vi "get_length_or_depth.vi"(8 "error in (no error)":errorcluster, 11 "ImageCollection in":refnum<class "ImageCollection.lvclass">) -> (0 "error out":errorcluster, 1 "total z depth":dbl[unit], 2 "movie length":dbl[unit], 3 "ImageCollection out":refnum<class "ImageCollection.lvclass">, 4 "type":T1)   [LabVIEW 2010, in "ImageCollection.lvclass"]
uses:
  ImageCollection.lvclass
  type_enum.ctl
  ImageCollection.lvclass/ImageCollection.ctl
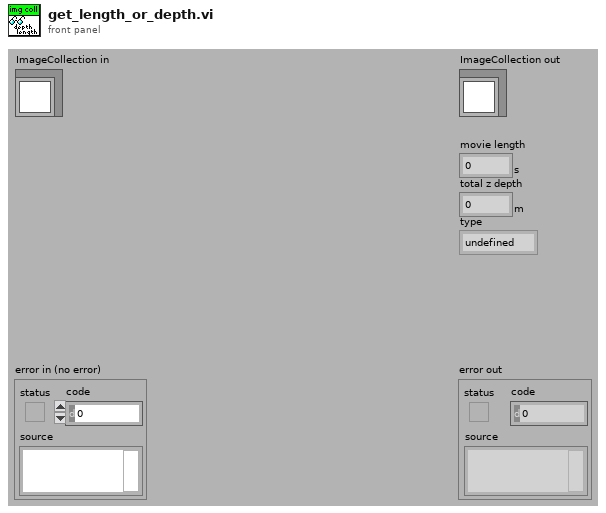
[diagram p1: front panel]
types:
  T1 = typedef "type_enum.ctl" = enum16{"undefined", "movie", "z-stack"}
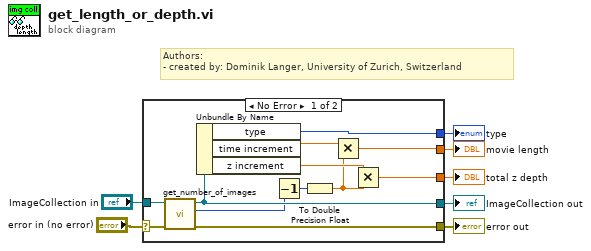
[diagram p0: block diagram]
diagram:
  # "Authors: \n- created by: Dominik Langer, University of Zurich, Switzerland"
  n1 = case shown="No Error" "error in (no error)" {
    selector: "error in (no error)" -> [w19 w21]
    tunnel: [w18 w21] -> w6
    tunnel: [w16 w20] -> w4
    tunnel: "ImageCollection in" -> [w17 w20]
    tunnel: [w10 _] -> w3
    tunnel: [w9 _] -> w2
    tunnel: [w8 _] -> w1
    frame No Error {
      n2 = call-dynamic "get_number_of_images.vi"("error in (no error)"=w19, "ImageCollection in"=w17) -> ("error out"=w18:errorcluster, "size"=w14:i32, "ImageCollection out"=w16:refnum<class "ImageCollection.lvclass">)  [unwired: 7 in]
      n3 = Unbundle By Name(w16) -> ("type"=w8:T1, "time increment"=w12:dbl[unit], "z increment"=w15:dbl[unit])
      n4 = Decrement(x=w14) -> (x-1=w13:i32)
      n5 = To Double Precision Float(number=w13) -> (double precision float=w11:dbl)
      n6 = Multiply(x=w12, y=w11) -> (x*y=w10:dbl[unit])
      n7 = Multiply(x=w15, y=w11) -> (x*y=w9:dbl[unit])
    }
    frame Error {
    }
  }
  "error out" <- w6
  "ImageCollection out" <- w4
  "movie length" <- w3
  "total z depth" <- w2
  "type" <- w1
